vi "GetSyncBdcstEvents.vi"(7 "error in (no error)":errorcluster) -> (3 "Event Registration Refnum":refnum<event-registration>, 5 "error out":errorcluster)   [LabVIEW 2018, in "Test.lvclass"]
uses:
  Test.lvclass
  Sync/SyncModule/Protected/clEventType.ctl
  Sync/SyncModule/SyncModule.lvlib
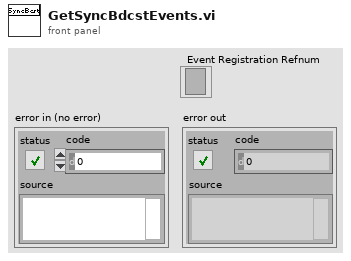
[diagram p1: front panel]
types:
  T1 = typedef "SyncModule.lvlib/clBroadcastEvents.ctl" = cluster{"DidInit":refnum<user-event>, "StatusUpdate":refnum<user-event>, "ErrorReport":refnum<user-event>, "DidStop":refnum<user-event>, "PathToINI":refnum<user-event>, "TriggerTime":refnum<user-event>, "LockStatus":refnum<user-event>, "Info":refnum<user-event>, "ClockProperties":refnum<user-event>}
  T2 = cluster{"TriggerTime":refnum<user-event>, "LockStatus":refnum<user-event>, "ErrorReport":refnum<user-event>, "Info":refnum<user-event>, "ClockProperties":refnum<user-event>}
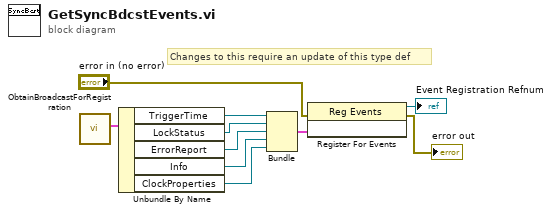
[diagram p0: block diagram]
diagram:
  # "Changes to this require an update of this type def"
  n1 = call "ObtainBroadcastForRegistration.vi"() -> ("SyncBroadcastEvents"=w10:T1)  [unwired: 10 in, 1 out]
  n2 = Unbundle By Name(w10) -> ("TriggerTime"=w9:refnum<user-event>, "LockStatus"=w8:refnum<user-event>, "ErrorReport"=w6:refnum<user-event>, "Info"=w5:refnum<user-event>, "ClockProperties"=w2:refnum<user-event>)
  n3 = Bundle("TriggerTime"=w9, "LockStatus"=w8, "ErrorReport"=w6, "Info"=w5, "ClockProperties"=w2) -> (w7:T2)  [unwired: 1 in]
  n4 = register-events(error in="error in (no error)", w7) -> (reference out=→"Event Registration Refnum":refnum<event-registration>, error out=→"error out":errorcluster)  [unwired: 1 in]
